vi "HumanNetwork.vi"(8 "error in (no error)":errorcluster) -> (0 "error out":errorcluster)   [LabVIEW 2020]
doc: "Human Network\n\nInput\n --Error in \n\nOutput\n --Error out"
uses:
  HumanGlobal.vi
  <vilib>/Rock Robotics/Network Tables/NT Write Boolean.vi
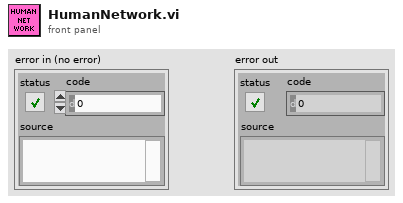
[diagram p1: front panel]
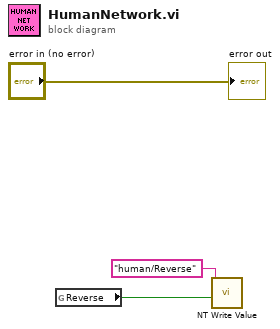
[diagram p0: block diagram]
diagram:
  n1 = global read "HumanGlobal.vi" "Reverse"() -> (w2:bool)
  n2 = call-poly <vilib>:"NT Write Value.vi"("value"=w2, "name"="human/Reverse") -> ()  [unwired: 9 in, 1 out]
  "error out" <- "error in (no error)"
